vi "Interframe_template-matched-tempbox_displacements_Checked_VI_2.vi"() -> ()   [LabVIEW 2012]
uses:
  <vilib>/Utility/file.llb/Write To Spreadsheet File (I64).vi
  <vilib>/imath/engines/lvmath2/RunTimeEngine/NodeEndStatement/NIMS_NodeEndStatement_Output.vi
  <instcachedir>/0/NIMS_NodeEndStatement_Output_53EC0D466D134D7ABD903AC30B43404B.lvgen/NIMS_NodeEndStatement_Output_53EC0D466D134D7ABD903AC30B43404B_004.vi
  <vilib>/imath/engines/lvmath2/RunTimeEngine/ErrorHandling/NIMS_Finalize Error.vi
panel:
  in  "Template \n      in \n1st frame\n    e_z":u16=291
  in  "Template \n      in \n1st frame\n    e_x":u16=692
  in  "Template \n      in \n1st frame\n    s_z":u16=282
  in  "Template \n      in\n1st frame\n     s_x":u16=658
  out "Template in 1st frame of every iteration":u8[][](array[numeric])
  out "Frames":T1(plugin-control)
  out "Frame\nDelta_X\nDelta_Z":i16[][](array[numeric])
  out "Matched TempBox (z,x): ROI-Frame_of_Reference":u8[][](array[numeric])
  out "Min_SAD":u16[](array[numeric])
  out "Delta_Z (TempBox-Template)":i16[](array[numeric])
  out "Delta_X (TempBox-Template)":i16[](array[numeric])
  out "SAD":u32[][](array[numeric])
  out "SAD_1Darray":u32[](array[numeric])
  in  "ROI in\n2nd frame\n    e_z":u16=301
  in  "ROI in\n2nd frame\n    s_z":u16=272
  in  "ROI in\n2nd frame\n    e_x":u16=727
  in  "ROI in\n2nd frame\n    s_x":u16=623
  in  "?":bool
  in  "1st frame":u16=153
  in  "Last frame":u16=154
  out "framesPerSecond":u16
  out "Image Type":T2 items=["Grayscale (U8)", "Grayscale (I16)", "Grayscale (SGL)", "Complex (CSG)", "RGB (U32)", "HSL (U32)", "RGB (U64)"]
  out "Number of Frames":u16
  in  "Path":path=path "C:/Users/admin/Desktop/lohit/pat3.avi"
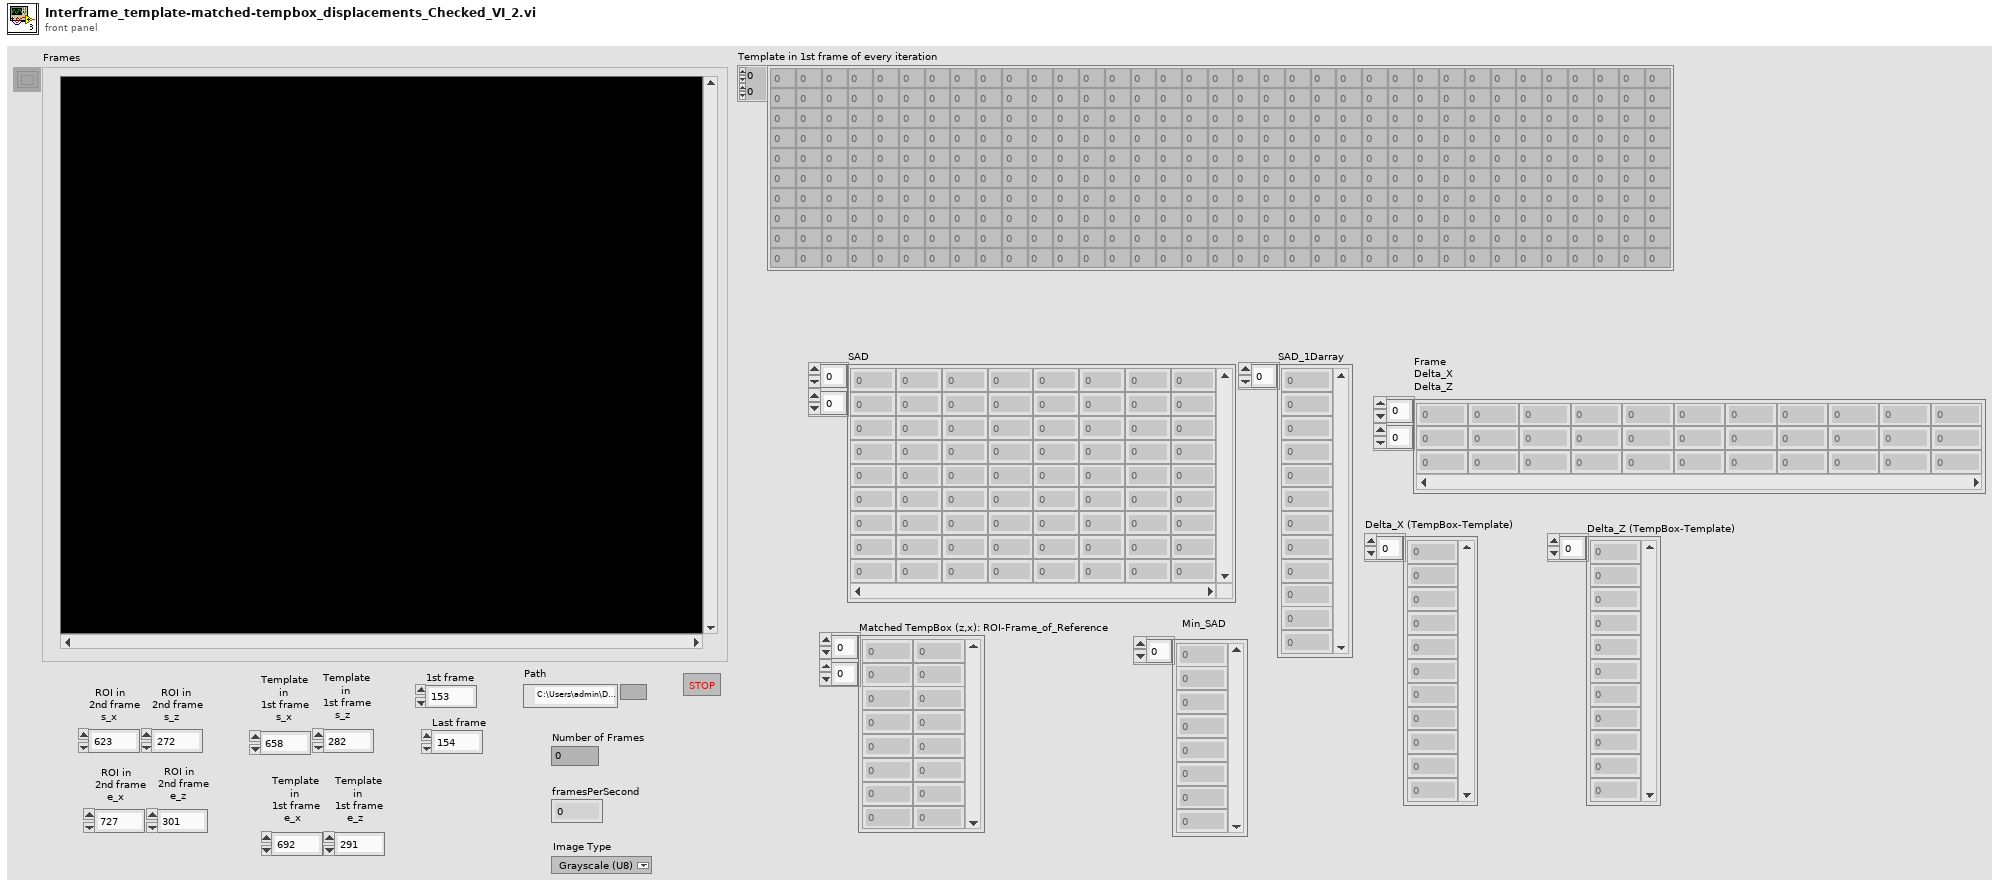
[diagram p1: front panel]
types:
  T1 = typedef "IMAQ Image.ctl" = refnum<image>
  T2 = typedef "Image Type" = u32
  T3 = typedef "AviRefnum.ctl" = refnum<k1>
  T4 = cluster{"width":u32, "height":u32, "framesPerSecond":u32, "compressionFilter":string, "hasData":bool}
  T5 = cluster{"[0]":u8, "[1]":u8, "[2]":u8, "[3]":u8, "[4]":u8, "[5]":u8, "[6]":u8, "[7]":u8, "[8]":u8}
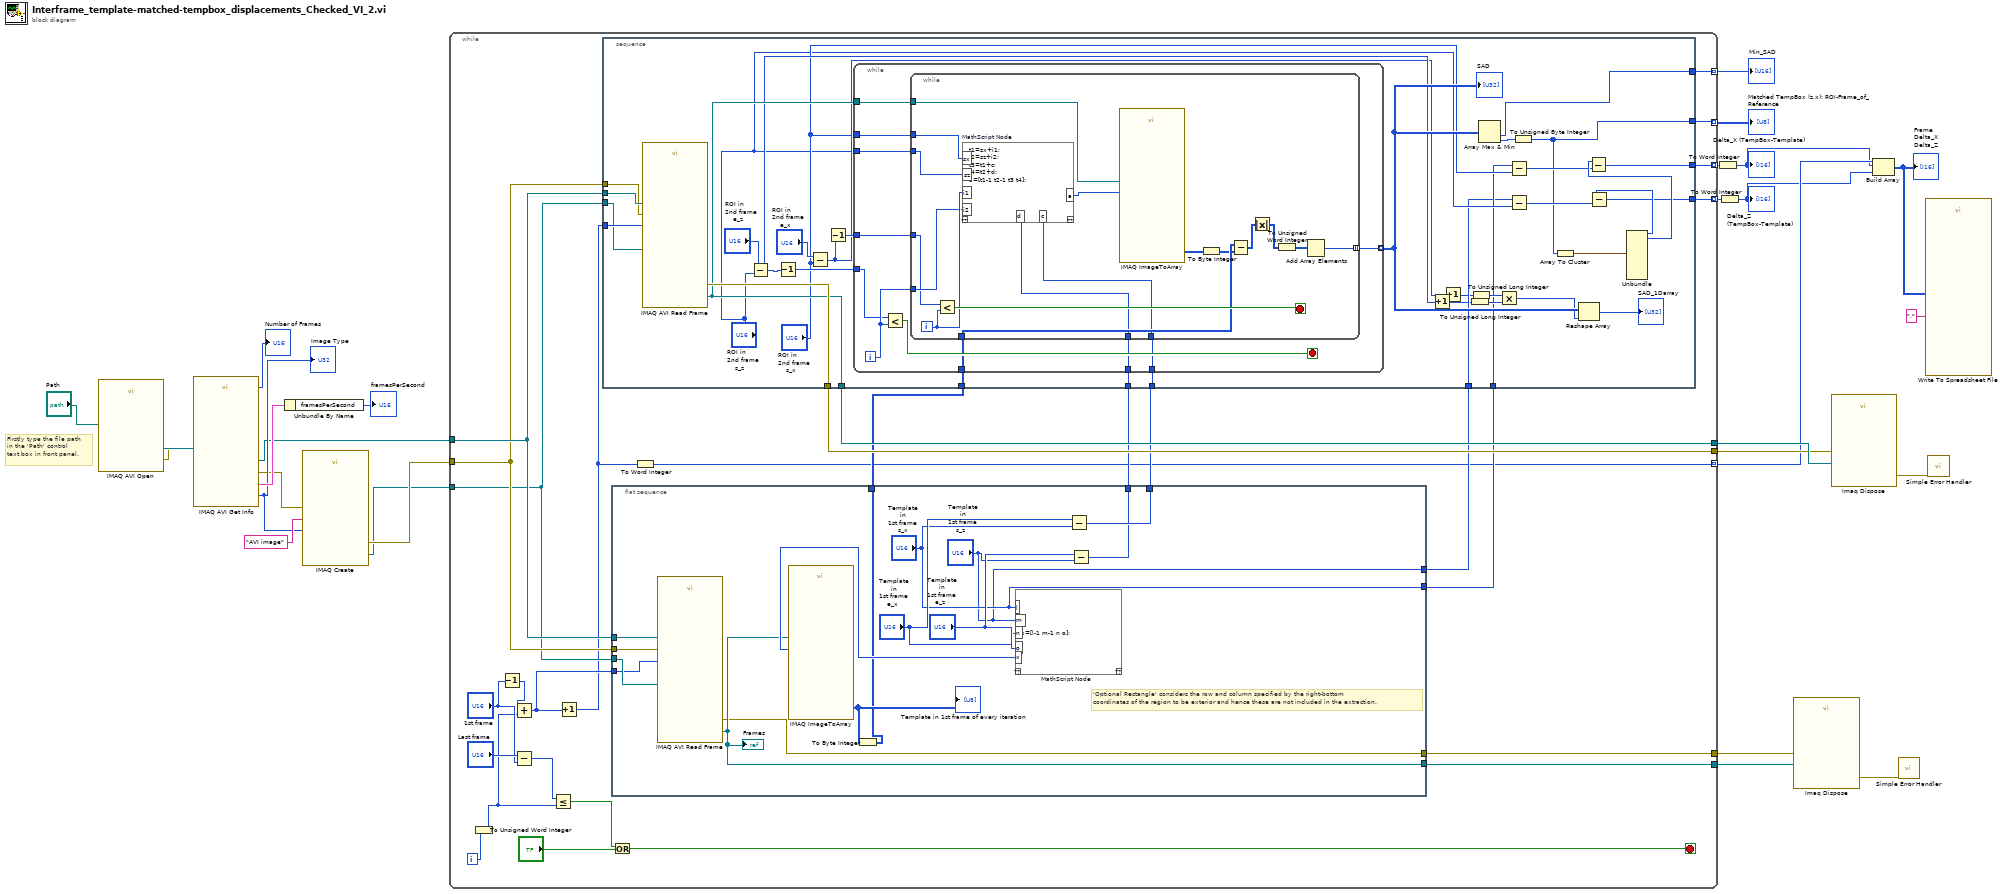
[diagram p0: block diagram]
diagram:
  # "Firstly type the file path\nin the 'Path' control \ntext box in front panel."
  n1 = call "IMAQ AVI Open"("AVI Path"="Path") -> ("error out"=w20:errorcluster, "Avi Refnum"=w26:T3)  [unwired: 9 in]
  n2 = call "IMAQ AVI Get Info"("error in (no error)"=w20, "Avi Refnum"=w26) -> ("error out"=w19:errorcluster, "Image Type"=w22:T2, "Number of Frames"=→"Number of Frames":u32, "Avi Refnum (duplicate)"=w18:T3, "Frame Data"=w24:T4)  [unwired: 5 in]
  "Image Type" <- w22
  n3 = Unbundle By Name(w24) -> ("framesPerSecond"=→"framesPerSecond":u32)
  n4 = call "IMAQ Create"("Image Name"="AVI image", "Image Type"=w22, "error in (no error)"=w19) -> ("New Image"=w16:T1, "error out"=w17:errorcluster)  [unwired: 2 in]
  n5 = while {
    tunnel: w18 -> [w41]
    tunnel: w17 -> [w40]
    tunnel: w16 -> [w39]
    tunnel: [w54] -> w14
    tunnel: [w53] -> w13
    tunnel: [w52] -> w10 mode=indexing
    tunnel: [w51] -> w9 mode=indexing
    tunnel: [w50] -> w7 mode=indexing
    tunnel: [w47] -> w8 mode=indexing
    tunnel: [w28] -> w11 mode=indexing
    tunnel: [w36] -> w6
    tunnel: [w35] -> w5
    i -> [w44]
    stop <- w55 stop-if-true
    n6 = To Unsigned Word Integer(number=w44) -> (unsigned 16bit integer=w29:u16)
    n7 = Decrement(x="1st frame") -> (x-1=w46:u16)
    n8 = Add(x=w46, y=w29) -> (x+y=w38:u16)
    n9 = Subtract(x="Last frame", y="1st frame") -> (x-y=w48:u16)
    n10 = Less Or Equal?(x=w48, y=w29) -> (x <= y?=w42:bool)
    n11 = Increment(x=w38) -> (x+1=w37:u16)
    n12 = stacked-sequence {
      tunnel: w41 -> [w136]
      tunnel: w40 -> [w134]
      tunnel: w39 -> [w135]
      tunnel: w37 -> [w137]
      tunnel: [w132] -> w54
      tunnel: [w133] -> w53
      tunnel: [w128] -> w52
      tunnel: [w127] -> w51
      tunnel: [w126] -> w50
      tunnel: [w105] -> w47
      tunnel: w34 -> [w110]
      tunnel: w31 -> [w109]
      tunnel: w30 -> [w108]
      tunnel: w33 -> [w107]
      tunnel: w32 -> [w106]
      frame #0 {
        n13 = call "IMAQ AVI Read Frame"("error in (no error)"=w134, "Frame Number"=w137, "Image"=w135, "Avi Refnum"=w136) -> ("error out"=w133:errorcluster, "Image Out"=w132:T1)  [unwired: 4 in, 2 out]
        n14 = Subtract(x="ROI in\n2nd frame\n    e_z", y="ROI in\n2nd frame\n    s_z") -> (x-y=w118:u16)
        n15 = Decrement(x=w118) -> (x-1=w119:u16)
        n16 = Subtract(x="ROI in\n2nd frame\n    e_x", y="ROI in\n2nd frame\n    s_x") -> (x-y=w115:u16)
        n17 = Decrement(x=w115) -> (x-1=w116:u16)
        n18 = while {
          tunnel: w132 -> [w147]
          tunnel: w110 -> [w145]
          tunnel: w107 -> [w144]
          tunnel: w106 -> [w143]
          tunnel: [w142] -> w124 mode=indexing
          tunnel: w119 -> [w141]
          tunnel: w116 -> [w140]
          tunnel: "ROI in\n2nd frame\n    s_x" -> [w139]
          tunnel: "ROI in\n2nd frame\n    s_z" -> [w138]
          i -> [w146]
          stop <- w148 stop-if-true
          n19 = Less?(x=w141, y=w146) -> (x < y?=w148:bool)
          n20 = while {
            tunnel: w147 -> [w163]
            tunnel: w146 -> [w161]
            tunnel: w145 -> [w156]
            tunnel: w144 -> [w154]
            tunnel: w143 -> [w153]
            tunnel: [w152] -> w142 mode=indexing
            tunnel: w140 -> [w151]
            tunnel: w139 -> [w150]
            tunnel: w138 -> [w149]
            i -> [w162]
            stop <- w164 stop-if-true
            n21 = Less?(x=w151, y=w162) -> (x < y?=w164:bool)
            n22 = mathscript code="t1=sx+i1;\nt2=sz+i2;\nt3=t1+c;\nt4=t2+d;\na=[t1-1 t2-1 t3 t4];"("sx"=w150, "sz"=w149, "i1"=w162, "i2"=w161, "c"=w154, "d"=w153) -> ("a"=w160:i32[])  [unwired: 1 in, 1 out]
            n23 = call "IMAQ ImageToArray"("Optional Rectangle"=w160, "Image"=w163) -> ("Image Pixels (U8)"=w165:u8[][])  [unwired: 2 in, 4 out]
            n24 = To Byte Integer(number=w165) -> (8bit integer=w155:i8[][])
            n25 = Subtract(x=w156, y=w155) -> (x-y=w158:i8[][])
            n26 = Absolute Value(x=w158) -> (abs(x)=w157:i8[][])
            n27 = To Unsigned Word Integer(number=w157) -> (unsigned 16bit integer=w159:u16[][])
            n28 = Add Array Elements(numeric array=w159) -> (sum=w152:u16)
          }
        }
        "SAD" <- w124
        n29 = Increment(x=w118) -> (x+1=w103:u16)
        n30 = Increment(x=w115) -> (x+1=w102:u16)
        n31 = To Unsigned Long Integer(number=w103) -> (unsigned 32bit integer=w121:u32)
        n32 = To Unsigned Long Integer(number=w102) -> (unsigned 32bit integer=w122:u32)
        n33 = Array Max & Min(array=w124) -> (min value=w126:u16, min index (indices)=w125:i32[])  [unwired: 2 out]
        n34 = Multiply(x=w122, y=w121) -> (x*y=w123:u32)
        n35 = Subtract(x=w109, y="ROI in\n2nd frame\n    s_x") -> (x-y=w113:u16)
        n36 = Subtract(x=w108, y="ROI in\n2nd frame\n    s_z") -> (x-y=w114:u16)
        n37 = To Unsigned Byte Integer(number=w125) -> (unsigned 8bit integer=w105:u8[])
        n38 = Array To Cluster(array=w105) -> (cluster=w131:T5)
        n39 = Reshape Array "Reshape Array"(w124, w123) -> (→"SAD_1Darray":u16[])
        n40 = Unbundle "Unbundle"(w131) -> ("[0]"=w129:u8, "[1]"=w130:u8)  [unwired: 7 out]
        n41 = Subtract(x=w130, y=w113) -> (x-y=w128:u16)
        n42 = Subtract(x=w129, y=w114) -> (x-y=w127:u16)
      }
    }
    n43 = flat-sequence {
      tunnel: w41 -> [w67]
      tunnel: w40 -> [w66]
      tunnel: w39 -> [w65]
      tunnel: w38 -> [w64]
      tunnel: [w63] -> w36
      tunnel: [w62] -> w35
      tunnel: [w61] -> w34
      tunnel: [w59] -> w33
      tunnel: [w58] -> w32
      tunnel: ["Template \n      in\n1st frame\n     s_x"] -> w31
      tunnel: ["Template \n      in \n1st frame\n    s_z"] -> w30
      frame #0 {
        # "'Optional Rectangle' considers the row and column specified by the right-bottom\ncoordinates of the region to be exterior and hence these are not included in the extraction."
        n44 = call "IMAQ AVI Read Frame"("error in (no error)"=w66, "Frame Number"=w64, "Image"=w65, "Avi Refnum"=w67) -> ("error out"=w62:errorcluster, "Image Out"=w63:T1)  [unwired: 4 in, 2 out]
        "Frames" <- w63
        n45 = mathscript code="x=[l-1 m-1 n o];"("l"="Template \n      in\n1st frame\n     s_x", "m"="Template \n      in \n1st frame\n    s_z", "n"="Template \n      in \n1st frame\n    e_x", "o"="Template \n      in \n1st frame\n    e_z") -> ("x"=w69:i32[])  [unwired: 1 in, 1 out]
        n46 = call "IMAQ ImageToArray"("Optional Rectangle"=w69, "Image"=w63) -> ("Image Pixels (U8)"=w70:u8[][])  [unwired: 2 in, 4 out]
        "Template in 1st frame of every iteration" <- w70
        n47 = To Byte Integer(number=w70) -> (8bit integer=w61:i8[][])
        n48 = Subtract(x="Template \n      in \n1st frame\n    e_x", y="Template \n      in\n1st frame\n     s_x") -> (x-y=w59:u16)
        n49 = Subtract(x="Template \n      in \n1st frame\n    e_z", y="Template \n      in \n1st frame\n    s_z") -> (x-y=w58:u16)
      }
    }
    n50 = Or(x=w42, y="?") -> (x .or. y?=w55:bool)
    n51 = To Word Integer(number=w37) -> (16bit integer=w28:i16)
  }
  "Min_SAD" <- w7
  "Matched TempBox (z,x): ROI-Frame_of_Reference" <- w8
  n52 = To Word Integer(number=w10) -> (16bit integer=w1:i16[])
  "Delta_X (TempBox-Template)" <- w1
  n53 = To Word Integer(number=w9) -> (16bit integer=w2:i16[])
  "Delta_Z (TempBox-Template)" <- w2
  n54 = call "Imaq Dispose"("Image"=w6, "error in (no error)"=w5) -> ("error out"=w12:errorcluster)  [unwired: 4 in]
  n55 = call "Imaq Dispose"("Image"=w14, "error in (no error)"=w13) -> ("error out"=w15:errorcluster)  [unwired: 4 in]
  n56 = Build Array(w11, w1, w2) -> (w3:i16[][])
  "Frame\nDelta_X\nDelta_Z" <- w3
  n57 = call <vilib>:"Simple Error Handler.vi"("error in (no error)"=w12) -> ()  [unwired: 4 in, 5 out]
  n58 = call-poly <vilib>:"Write To Spreadsheet File.vi"("delimiter (\\t)"="," ("delimiter (\\t)"), "2D data"=w3) -> ()  [unwired: 6 in, 1 out]
  n59 = call <vilib>:"Simple Error Handler.vi"("error in (no error)"=w15) -> ()  [unwired: 4 in, 5 out]
